vi "Calculate_(101)-(11)_Local_Cost_F()-1.vi"(4 "[IN] Dot matrix with statuses \nfor potentially moving dots":i16[][](array[numeric]), 5 "[IN] Still connected\ntracks in group":T1, 6 "[IN] Potentially\nMoving (X,Y)":dbl[][](array[numeric]), 7 "[IN] Subtracks":T2(array[cluster]), 8 "error IN":errorcluster, 9 "[IN] Areas particles\nPrimary Detected":dbl[][](array[numeric]), 10 "[IN] Primary \n(X,Y) Detected":dbl[][](array[numeric]), 11 "[IN] Cost function":i8[](array[numeric])) -> (0 "error OUT":errorcluster, 3 "[OUT] Cost function":i8[](array[numeric]))   [LabVIEW 2013]
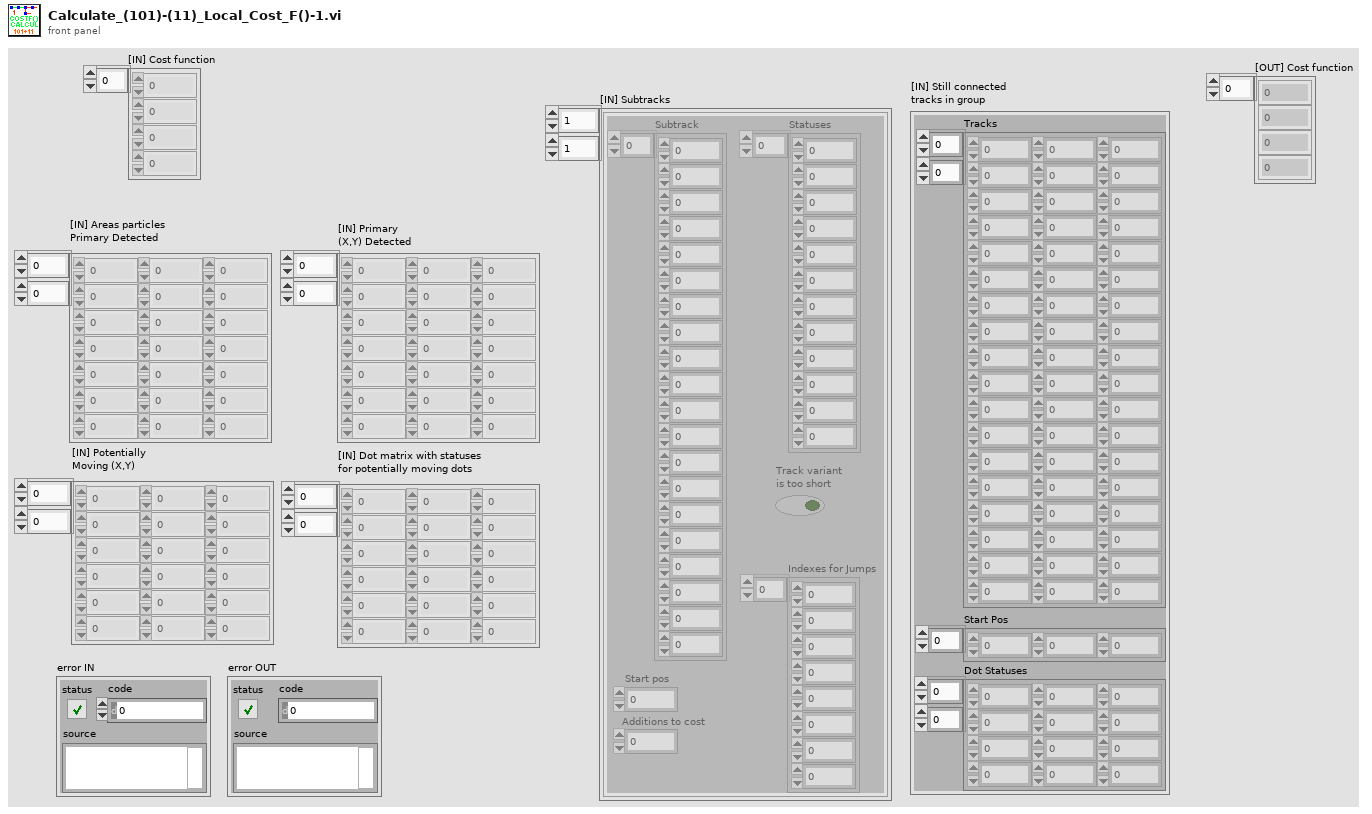
[diagram p1: front panel]
types:
  T1 = cluster{"Tracks":dbl[][], "Start Pos":i32[], "Dot Statuses":i16[][]}
  T2 = cluster{"Subtrack":dbl[], "Statuses":i16[], "Start pos":i32, "Additions to cost":i32, "Track variant \nis too short":bool, "Indexes for Jumps":i32[]}[][]
  T3 = cluster{"Subtrack":dbl[], "Statuses":i16[], "Start pos":i32, "Additions to cost":i32, "Track variant \nis too short":bool, "Indexes for Jumps":i32[]}[]
  T4 = cluster{"Subtrack":dbl[], "Statuses":i16[], "Start pos":i32, "Additions to cost":i32, "Track variant \nis too short":bool, "Indexes for Jumps":i32[]}
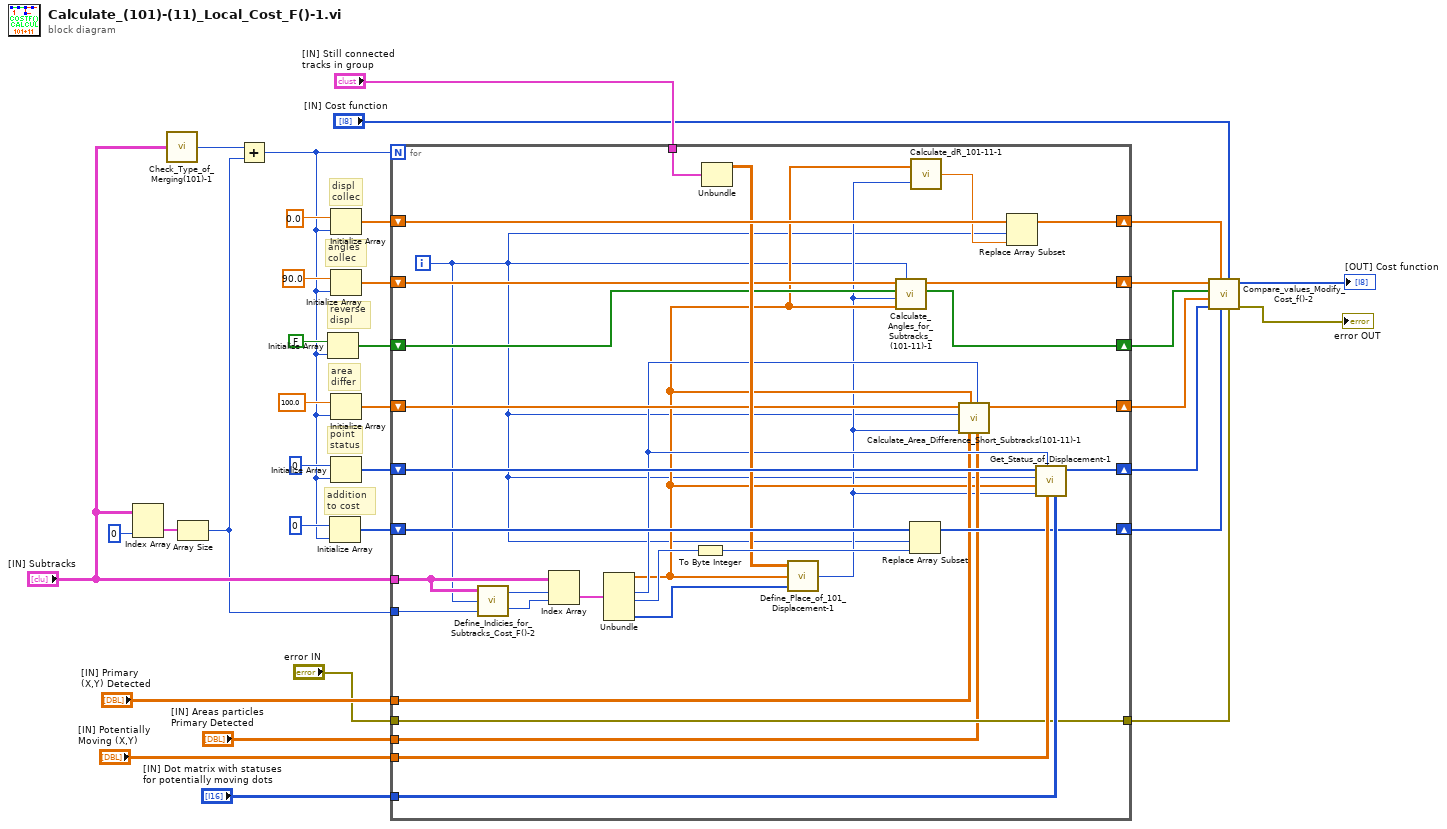
[diagram p0: block diagram]
diagram:
  # "addition \nto cost"
  # "point\nstatus"
  # "area \ndiffer"
  # "reverse \ndispl"
  # "angles \ncollec"
  # "displ \ncollec"
  n1 = Index Array(array="[IN] Subtracks", index (col)=0 ("disabled index (col)")) -> (element=w20:T3)  [unwired: 1 in]
  n2 = call "Check_Type_of_Merging(101)-1.vi"("[IN] Subtracks"="[IN] Subtracks") -> ("[OUT] # of Additional Costs"=w3:i32)
  n3 = Array Size(array=w20) -> (size(s)=w2:i32)
  n4 = Add(x=w3, y=w2) -> (x+y=w1:i32)
  n5 = Initialize Array(FALSE, w1) -> (w29:bool[])
  n6 = Initialize Array(i8 0, w1) -> (w23:i8[])
  n7 = Initialize Array(0.0, w1) -> (w33:dbl[])
  n8 = Initialize Array(90.0, w1) -> (w31:dbl[])
  n9 = Initialize Array(100.0, w1) -> (w27:dbl[])
  n10 = Initialize Array(i16 0, w1) -> (w25:i16[])
  n11 = for {
    N: w1 -> [_]
    tunnel: "[IN] Subtracks" -> [w39]
    tunnel: "[IN] Still connected\ntracks in group" -> [w65]
    shift-right: [w63] -> w10
    shift-left: w33 -> [w64]
    shift-right: [w49] -> w14
    shift-left: w31 -> [w50]
    shift-right: [w47] -> w13
    shift-left: w29 -> [w48]
    tunnel: "[IN] Primary \n(X,Y) Detected" -> [w44]
    tunnel: "[IN] Areas particles\nPrimary Detected" -> [w43]
    shift-right: [w42] -> w12
    shift-left: w27 -> [w46]
    tunnel: "[IN] Potentially\nMoving (X,Y)" -> [w61]
    tunnel: "[IN] Dot matrix with statuses \nfor potentially moving dots" -> [w60]
    shift-right: [w59] -> w11
    shift-left: w25 -> [w62]
    shift-right: [w55] -> w8
    shift-left: w23 -> [w58]
    tunnel: "error IN" -> [w54]
    tunnel: [w54] -> w6
    tunnel: w2 -> [w37]
    i -> [w38]
    n12 = call "Define_Indicies_for_Subtracks_Cost_F()-2.vi"("[IN] Number of Rows"=w37, "[IN] Current index"=w38, "[IN] Subtracks"=w39) -> ("[OUT] Column \n# for Subtrack"=w35:i32, "[OUT] Row # \nfor Subtrack"=w36:i32)
    n13 = Index Array(array=w39, index (row)=w36, index (col)=w35) -> (element=w66:T4)
    n14 = Unbundle(w66) -> ("Subtrack"=w41:dbl[], "Start pos"=w45:i32, "Additions to cost"=w57:i32, "Indexes for Jumps"=w52:i32[])  [unwired: 2 out]
    n15 = To Byte Integer(number=w57) -> (8bit integer=w56:i8)
    n16 = Unbundle(w65) -> ("Tracks"=w53:dbl[][])  [unwired: 2 out]
    n17 = call "Define_Place_of_101_Displacement-1.vi"("[IN] Indexes for Jumps"=w52, "[IN] Subtrack"=w41, "[IN] Tracks"=w53) -> ("[OUT] Index of \"11\" Dis\nplacement in Subtrack"=w40:i32)  [unwired: 2 in]
    n18 = call "Calculate_Angles_for_Subtracks_(101-11)-1.vi"("[IN] Index of subtrack"=w38, "[IN] Subtrack"=w41, "[IN] Index of \"101\" Dis-\nplacement in Subtrack"=w40, "[IN] Reverse Displ or Not"=w48, "[IN] Array with Angles \nBetween Displacement"=w50) -> ("[OUT] Reverse displacement or not"=w47:bool[], "[OUT] Angles betwe\nen two displacements"=w49:dbl[])  [unwired: 3 in]
    n19 = Replace Array Subset(array=w58, new element=w56, index=w38) -> (w55:i8[])
    n20 = call "Calculate_dR_101-11-1.vi"("[IN] Index of \"101\"\nDisplacement"=w40, "[IN] Subtrack"=w41) -> ("[OUT] Displacement average"=w51:dbl)
    n21 = call "Calculate_Area_Difference_Short_Subtracks(101-11)-1.vi"("[IN] Areas particles\nPrimary Detected"=w43, "[IN] Start pos"=w45, "[IN] Primary \n(X,Y) Detected"=w44, "[IN] Subtrack"=w41, "[IN] Index of \"101\" Dis-\nplacement in Subtrack"=w40, "[IN] Index of\n subtrack"=w38, "[IN] Areas \ndifference"=w46) -> ("[OUT] Areas differen\nce (101 + 11 points)"=w42:dbl[])  [unwired: 4 in]
    n22 = Replace Array Subset(array=w64, new element=w51, index=w38) -> (w63:dbl[])
    n23 = call "Get_Status_of_Displacement-1.vi"("[IN] Dot matrix with statuses\nfor potentially moving dots"=w60, "[IN] Potentially\nMoving (X,Y)"=w61, "[IN] Start pos"=w45, "[IN] Index of Problem\nPoint in Subtrack"=w40, "[IN] Subtrack"=w41, "[IN] Index of\n subtrack"=w38, "[IN] Displace-\nment Statuses"=w62) -> ("[OUT] Displace\nment Statuses"=w59:i16[])  [unwired: 4 in]
  }
  n24 = call "Compare_values_Modify_Cost_f()-2.vi"("error IN"=w6, "[IN] Cost function"="[IN] Cost function", "[IN] Additions to cost"=w8, "[IN] Array of displa\ncement differences"=w10, "[IN] Statuses of points"=w11, "[IN] Areas \ndifferences"=w12, "[IN] Reverse or not"=w13, "[IN] Angles betwe\nen displacements"=w14) -> ("error OUT"=→"error OUT":errorcluster, "[OUT] Cost function"=→"[OUT] Cost function":i8[])  [unwired: 2 in]
